vi "Construct Connection.vi"(10 "destination":string, 11 "source":string) -> (3 "Connection":T1)   [LabVIEW 2017, in "Switch Scripting.lvlib"]
uses:
  Switch Scripting.lvlib
  Connection.ctl
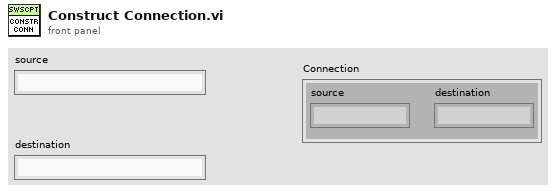
[diagram p1: front panel]
types:
  T1 = typedef "Switch Scripting.lvlib/Connection.ctl" = cluster{"source":string, "destination":string}
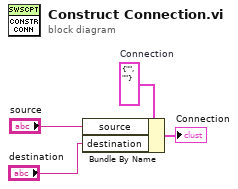
[diagram p0: block diagram]
diagram:
  w1 = T1 {"source"="", "destination"=""}  # Connection
  n1 = Bundle By Name(cluster=w1, "source"="source", "destination"="destination") -> (→"Connection":T1)
